vi "AlliGator 1-Exp + IRF Fit v2.vi"(0 "Decay":cluster{"t Array":dbl[], "Data Array":dbl[]}, 5 "IRF":cluster{"t Array":dbl[], "IRF Array":dbl[]}, 7 "Fit Options":T9={"Show Fit Residuals"=TRUE, "Fit Model"=enum."1-Exponential", "Residual Type"=enum."Standard", "Max Decay Percentile"=0.0, "Min Decay Percentile"=0.0, "Show Full Decay"=TRUE, "Weights"=enum."Unweighted", "Fitting Method"=enum."Least Square", "Compute Parameter Uncertainties"=TRUE, "Periodic Boundaries"=TRUE, "Model Calculation"=enum."Simulation", "Period"=1.2500000000000001e-08, "Termination Criteria"={"Max Iterations"=1000, "Max Function Calls"=0, "Max Time"=1000.0, "Function Tolerance"=1e-06, "Parameter Tolerance"=1e-06, "Gradient Tolerance"=0.0, "Min Lambda"=1e-06, "Max Lambda"=1e-06, "Initial Tick Count"=0}, "Offset Resolution"=1.2500000000000001e-08, "Use Local IRF"=TRUE, "Fitting Algorithm"=enum."Levenberg-Marquardt"} {"Offset Resolution" min=0.0; "Period" min=0.0; "Min Decay Percentile" min=0.0 max=1.0; "Max Decay Percentile" min=0.0 max=1.0}, 11 "error in (no error)":errorcluster, 12 "parameter bounds":T8) -> (4 "Fitted Decay":cluster{"t Array":dbl[], "Fitted Array":dbl[]}, 6 "Residuals":cluster{"t Array":dbl[], "Residual Array":dbl[]}, 8 "Fit Output":T2={"best nonlinear fit"=[], "best fit parameters"=[], "R^2"=0.0, "RMSE"=0.0, "error out"={"status"=FALSE, "code"=0, "source"=""}, "Fitting Method"=enum."Least Square", "number of function calls"=0, "number of iterations"=0, "covariance"=[], "Chi 2"=0.0, "DOF"=0, "Fit Convergence Criterion"=enum."Continue", "Fitting Algorithm"=enum."Levenberg-Marquardt", "Weighted Fit"=FALSE, "Gradient"=0.0, "|Delta Chi 2|"=0.0, "|Delta Chi 2|/Chi 2"=0.0, "Max |Delta a| /|a|"=0.0, "Lambda"=-1.0, "RSS"=0.0, "AIC"=0.0, "BIC"=0.0, "Max number of function calls"=0, "Max number of iterations"=0, "IRF"={"X Array"=[], "Y Array"=[]}, "IRF Normalization Factor"=0.0, "Decay Normalization Factor"=0.0}, 10 "Delta Best Fit Parameters":dbl[](array[numeric]), 13 "Guess Parameters Options":T1=enum."User-provided (normalized)", 14 "Guess Parameters":dbl[](array[numeric]), 15 "error out":errorcluster)   [LabVIEW 2021, in "AlliGator Decay Analysis.lvlib" / "AlliGator Decay Fit.lvlib"]
doc: "Legacy code for 1-Exp decay fit."
uses:
  AlliGator Decay Fit.lvlib
  Fits/IRF(X)PSED/Decay Fit Options v2.ctl
  Fits/Decay Convolution/Decay Model.ctl
  Fits/Residual Type.ctl
  Fits/IRF(X)PSED/Fit Weights Type.ctl
  Fits/Non-linear Fitting Method v2.ctl
  Fits/Fit Calculation Method.ctl
  Fits/Non-linear Fitting Algorithm.ctl
  Fits/Non-linear Fit Output v3.ctl
  Fits/Nonlinear Fit Method.ctl
  <vilib>/Analysis/Matrix/Datatypes/RealMatrix.ctl
  Fits/Convergence Criteria.ctl
  Graphs/XY Graph/XY Plot Data.ctl
  AlliGator Guess Parameters Options.ctl
  AlliGator Settings List.ctl
  Fits/Decay Convolution/Fit Control Data.ctl
  AlliGator Variables List.ctl
  Fits/Decay Convolution/LM model function and gradient (1-Exp, Convolved) v2.vi
  Phasor/Phasor Abort Parallel Computation.vi
  Fits/Decay Convolution/LM model function and gradient (1-Exp, Convolved, Periodic) v3.vi
  Fits/Decay Convolution/LM model function and gradient (1-Exp, Gated, Periodic).vi
  <vilib>/Utility/error.llb/Error Cluster From Error Code.vi
  Fits/Abort Fit Global.vi
  <vilib>/ErrorRing/Error Ring.xnode
  Time/Time.lvlib
  Fits/Fits.lvlib
  AlliGator Settings.lvlib
  Phasor/Phasor.lvlib
  AlliGator Globals, Variables & Constants.lvlib
  Error/Error.lvlib
  Graphs/XY Graph/XY Graph Add-Ons.lvlib
  <vilib>/Analysis/Matrix/NI_Matrix.lvlib
panel:
  out "CPU (s)":dbl
  out "XY Graph":T15(graph)
  # "Offset\nBaseline\nAmplitude\nLifetime"
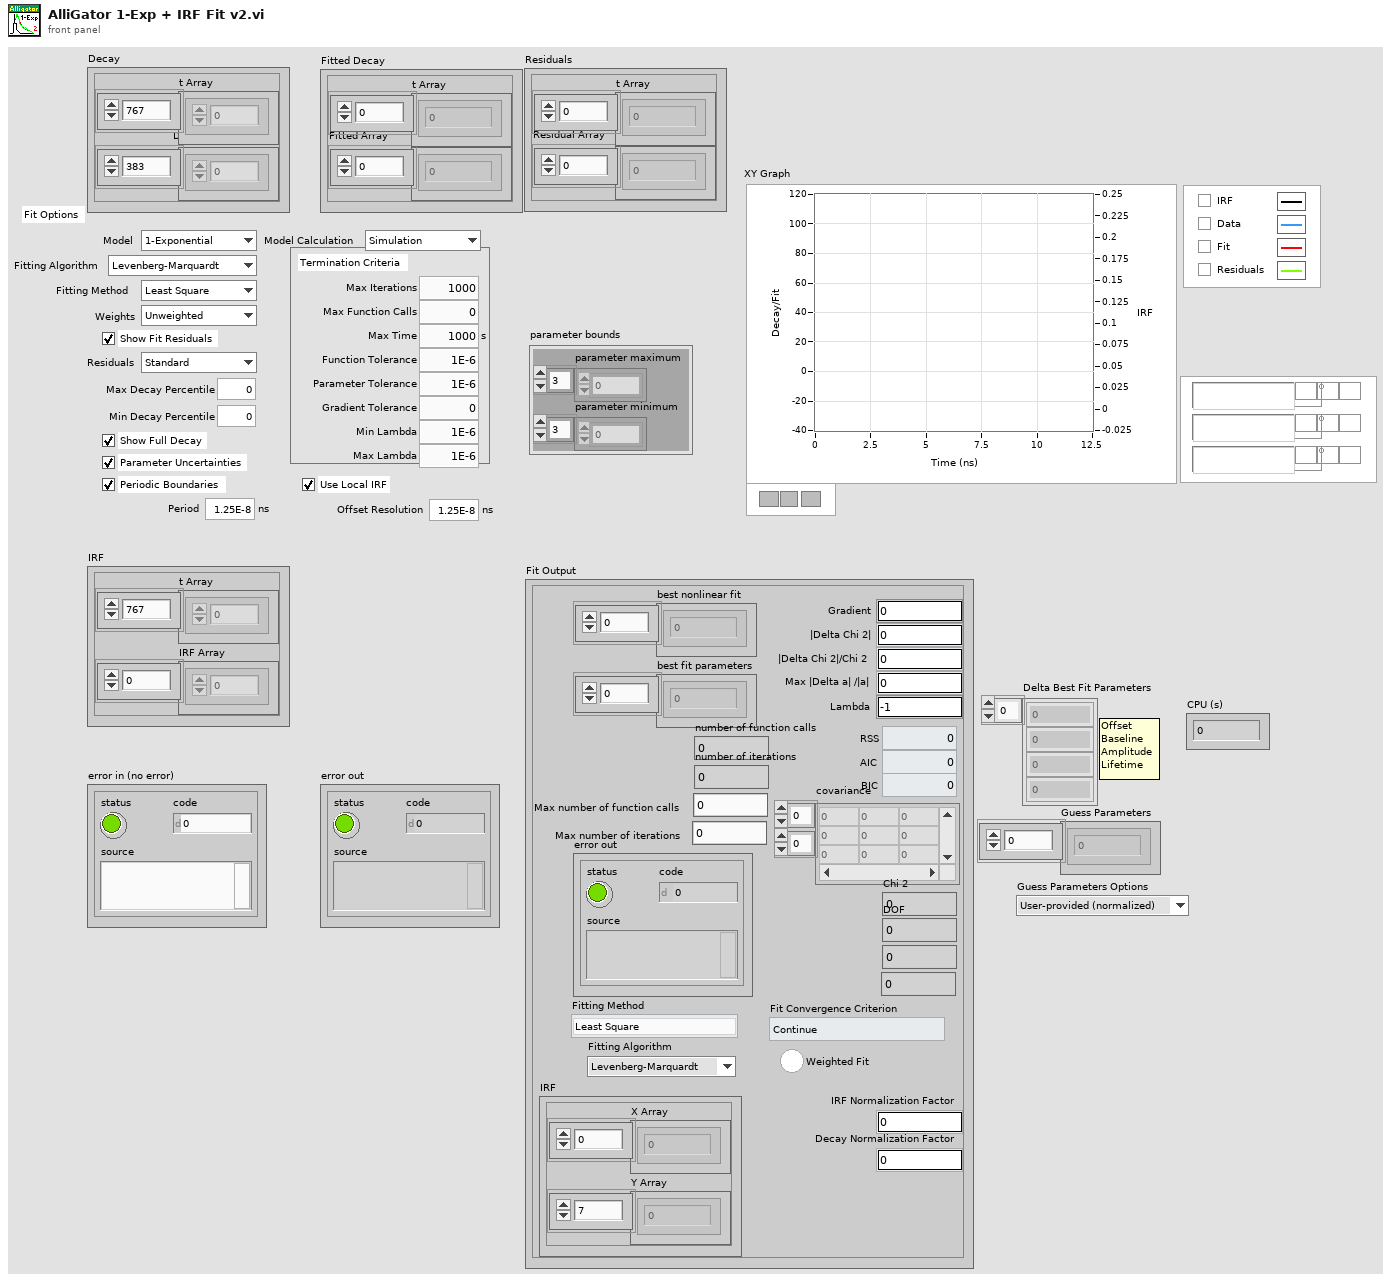
[diagram p1: front panel]
types:
  T1 = typedef "AlliGator Decay Analysis.lvlib/AlliGator Decay Fit.lvlib/AlliGator Guess Parameters Options.ctl" = enum16{"Numerically estimated", "User-provided", "User-provided (normalized)", "Last valid fitted parameters"}
  T2 = typedef "Fits.lvlib/Non-linear Fit Output v3.ctl" = cluster{"best nonlinear fit":dbl[], "best fit parameters":dbl[], "R^2":dbl, "RMSE":dbl, "error out":errorcluster, "Fitting Method":T3, "number of function calls":i32, "number of iterations":i32, "covariance":T4, "Chi 2":dbl, "DOF":i32, "Fit Convergence Criterion":T5, "Fitting Algorithm":T6, "Weighted Fit":bool, "Gradient":dbl, "|Delta Chi 2|":dbl, "|Delta Chi 2|/Chi 2":dbl, "Max |Delta a| /|a|":dbl, "Lambda":dbl, "RSS":dbl, "AIC":dbl, "BIC":dbl, "Max number of function calls":i32, "Max number of iterations":i32, "IRF":T7, "IRF Normalization Factor":dbl, "Decay Normalization Factor":dbl}
  T3 = typedef "Fits.lvlib/Nonlinear Fit Method.ctl" = enum16{"Least Square", "Least Absolute Residual", "Bisquare", "MLE"}
  T4 = typedef "NI_Matrix.lvlib/RealMatrix.ctl" = dbl[][]
  T5 = typedef "Fits.lvlib/Convergence Criteria.ctl" = enum16{"Continue", "Tolerances Exceeded", "Max Time Exceeded", "Max Iterations Exceeded", "Max Function Evaluations Exceeded", "Scale Range Exceeded"}
  T6 = typedef "Fits.lvlib/Non-linear Fitting Algorithm.ctl" = enum16{"Levenberg-Marquardt", "Trust-Region Dogleg"}
  T7 = typedef "XY Graph Add-Ons.lvlib/XY Plot Data.ctl" = cluster{"X Array":dbl[], "Y Array":dbl[]}
  T8 = cluster{"parameter minimum":dbl[], "parameter maximum":dbl[]}
  T9 = typedef "Fits.lvlib/Decay Fit Options v2.ctl" = cluster{"Show Fit Residuals":bool, "Fit Model":T10, "Residual Type":T11, "Max Decay Percentile":dbl, "Min Decay Percentile":dbl, "Show Full Decay":bool, "Weights":T12, "Fitting Method":T13, "Compute Parameter Uncertainties":bool, "Periodic Boundaries":bool, "Model Calculation":T14, "Period":dbl[unit], "Termination Criteria":cluster{"Max Iterations":i32, "Max Function Calls":i32, "Max Time":dbl[unit], "Function Tolerance":dbl, "Parameter Tolerance":dbl, "Gradient Tolerance":dbl, "Min Lambda":dbl, "Max Lambda":dbl, "Initial Tick Count":u32}, "Offset Resolution":dbl[unit], "Use Local IRF":bool, "Fitting Algorithm":T6}
  T10 = typedef "Fits.lvlib/Decay Model.ctl" = enum16{"1-Exponential", "2-Exponentials"}
  T11 = typedef "Fits.lvlib/Residual Type.ctl" = enum16{"Standard", "Normalized", "Reduced"}
  T12 = typedef "Fits.lvlib/Fit Weights Type.ctl" = enum16{"Unweighted", "1/Variance", "Best of All"}
  T13 = typedef "Fits.lvlib/Non-linear Fitting Method v2.ctl" = enum16{"Least Square", "Least Absolute Residual", "Bisquare", "MLE", "-", "Best of All"}
  T14 = typedef "Fits.lvlib/Fit Calculation Method.ctl" = enum16{"Simulation", "Convolution", "Integration"}
  T15 = cluster{"t Array":dbl[], "best nonlinear fit":dbl[]}[]
  T16 = typedef "AlliGator Settings.lvlib/AlliGator Settings List.ctl" = enum16{"GUI:Visible Settings Tab", "GUI:Last Run Version", "Source Image:Use Image Histogram for Contrast", "Source Image:Low Count Pixels Rejection Options", "Source Image:High Count Pixels Rejection Options", "Source Image:Use Image Brightness", "Source Image:Blend Overlay with Image Background", "Source Image:Use Fixed ROI Diameter", "Source Image:ROI Diameter", "Source Image:ROI Center Color", "Source Image:Peak Threshold", "Source Image:Intensity Threshold", "Source Image:Image Binning Options", "Source Image:Image Smoothing Options", "Source Image:Image Histogram Active", "Source Image:Invert Binary Mask", "Source Image:Hot Pixel Removal", "Source Image:Overlay Analyzed ROI Center", "Source Image:Auto-Adjust Contrast", "Source Image:Histogram Lower Percentile", "Source Image:Histogram Upper Percentile", "Source Image:Save Source Image", "Source Image:Scale Bar Options", "Source Image:Image Resolution (Pixel Size)", "Source Image:Flatfield Correction", "Source Image:Show Dead Left Columns Correction", "Source Image:Dead Left Columns Correction", "Source Image:Image Pre-Processing Operations Order", "Source Image:Overlay ROI Median", "Source Image:Median Overlay Color", "Data Information:Gate Width", "Data Information:Nanotime Gate Separation", "Data Information:Macrotime Gate Separation", "Data Information:Gate Step", "Data Information:# Gates", "Data Information:Gate Image Exposure", "Data Information:Gate Image Integration", "Data Information:Gates to Skip", "Data Information:Gates to Keep", "Data Information:Define Gates to", "Data Information:Channel Name", "Data Information:Available Channel Names", "Data Information:Channel Arithmetic", "Data Information:Background File Subtraction", "Data Information:Background File", "Data Information:Background Scaling Factor", "Data Information:Background Pile-up Correction", "Data Information:Background Pixel Well Capacity", "Data Information:Laser Period", "Data Information:SYNC Period", "Data Information:Pile-up Correction", "Data Information:Pixel Well Capacity", "Data Information:Dataset Scaling Factor", "Fluorescence Decay_Decay Pre-Processing:Reverse Gates", "Fluorescence Decay_Decay Pre-Processing:Verbose Decay Pre-Processing", "Fluorescence Decay_Decay Pre-Processing:Use Decay Pre-Processing", "Fluorescence Decay_Decay Pre-Processing:Background Subtraction", "Fluorescence Decay_Decay Pre-Processing:Background Definition Range", "Fluorescence Decay_Decay Pre-Processing:Baseline Subtraction Method", "Fluorescence Decay_Decay Pre-Processing:Decay Pre-Processing Operations Order", "Fluorescence Decay_Decay Pre-Processing:Smoothing Parameter", "Fluorescence Decay_Decay Pre-Processing:Shift Decay", "Fluorescence Decay_Decay Pre-Processing:Decay Shift Parameters", "Fluorescence Decay_Decay Pre-Processing:Fold Decay", "Fluorescence Decay_Decay Pre-Processing:# Folds", "Fluorescence Decay_Decay Pre-Processing:1-Normalize Decay", "Fluorescence Decay_Decay Pre-Processing:[0-1]-Normalize Decay", "Fluorescence Decay_Decay Pre-Processing:Smoothen Decay", "Fluorescence Decay_Decay Pre-Processing:Extrapolate Decay", "Fluorescence Decay_Decay Pre-Processing:Use Periodicity", "Fluorescence Decay_Decay Pre-Processing:Use Cursors", "Fluorescence Decay_Decay Pre-Processing:Tail Fraction", "Fluorescence Decay_Decay Pre-Processing:Head Fraction", "Fluorescence Decay_Decay Pre-Processing:Additional Points", "Fluorescence Decay_Decay Pre-Processing:Straighten Decay", "Fluorescence Decay_Decay Pre-Processing:Constant Background", "Fluorescence Decay_Decay Pre-Processing:Pixel-Normalize Decay", "Fluorescence Decay_Advanced Analysis:Extract IRF instead of Decay", "Fluorescence Decay_Advanced Analysis:IRF Extraction Options", "Fluorescence Decay_Advanced Analysis:IRF Optimization Options", "Fluorescence Decay_Advanced Analysis:Square Pulse Options", "Fluorescence Decay_Advanced Analysis:IRF Order", "Fluorescence Decay_Advanced Analysis:IRF Time Constants", "Fluorescence Decay_Advanced Analysis:Wavelet Analysis Options", "Fluorescence Decay_Advanced Analysis:Average Lifetime Options", "Fluorescence Decay_Fit Options:Fit Options", "Fluorescence Decay_Fit Options:Use Legacy Fitting Approach", "Fluorescence Decay_Fit Options:Use Data Information Laser Period", "Fluorescence Decay_Fit Parameters:Displayed Fit Parameters", "Fluorescence Decay_Fit Parameters:Fit Parameter Constraints", "Fluorescence Decay_Fit Parameters:Export Tabulated Results", "Fluorescence Decay_Fit Parameters:MLE Baseline Offset Type", "Fluorescence Decay_Fit Parameters:MLE Baseline Offset", "Fluorescence Decay_Fit Parameters:Guess Parameter Names", "Fluorescence Decay_Fit Parameters:Guess Parameter Values", "Fluorescence Decay_Fit Parameters:Guess Parameters Options", "Fluorescence Decay_Styles:Show Last Decay Only", "Fluorescence Decay_Styles:Decay Graph Color Array", "Fluorescence Decay:Decay Graph Active", "Fluorescence Decay Statistics:Min Peak Value", "Fluorescence Decay Statistics:Reject Low Decay Peak Pixels", "Fluorescence Decay Statistics:Reject High Decay Peak Pixels", "Fluorescence Decay Statistics:Max Peak Value", "Time Traces:Use File Timestamp", "Time Traces:Time Step", "Time Traces:Use Intensity Correction File", "Time Traces:Intensity Correction File", "Phasor Plot:Phasor Plot Smoothing Options", "Phasor Plot:Phasor Plot Size", "Phasor Plot:Phasor Plot Graphics Options", "Phasor Plot:Cumulative Phasor Plot", "Phasor Plot:Use Phasor Brightness", "Phasor Plot:Blend Overlay with Phasor Background", "Phasor Plot:Save Phasor Plot", "Phasor Plot:Show References", "Phasor Plot:Phasor Ratio Decay Range", "Phasor Plot:Exponential Fading", "Phasor Plot:Phasor Ratio Reference Colors", "Phasor Plot:Reference Radius", "Phasor Plot:Show Color Map Vertices", "Phasor Plot:Phasor Plot Active", "Phasor Plot:Phasor Ratio Color Map Type", "Phasor Plot:Phasor Ratio Color Map", "Phasor Plot:Phasor Ratio Display Range", "Phasor Plot:Selected Image ROI(s)", "Phasor Plot:All Image ROIs", "Phasor Plot:Selected Phasor Plot ROI(s)", "Phasor Plot:All Phasor Plot ROIs", "Phasor Plot:Phasor Ratio Color-Coded Quantity", "Phasor Plot:Store Phasor Harmonics", "Phasor Plot:Draw Reference Segment", "Phasor Plot:User-Defined Quantity", "Phasor Graph:Phasor Frequency", "Phasor Graph:Phasor Ratio Type", "Phasor Graph:Pixel-level Phasor Computation", "Phasor Graph:Save Phasor Graph", "Phasor Graph:Phasor Graph Active", "Phasor Graph:Phasor SDV Options", "Phasor Calibration:Use Backup Calibration if needed", "Phasor Graph:Define Shortest Lifetime as", "Phasor Calibration:Backup Calibration Type", "Phasor Calibration:Calibration Type", "Phasor Calibration:Calibration Lifetime", "Phasor Calibration:Calibration Map Algorithm", "Single-Exponential Phasor Locus (SEPL):Gate Parameters", "Single-Exponential Phasor Locus (SEPL):User-defined Gate", "Single-Exponential Phasor Locus (SEPL):User-defined IRF", "Single-Exponential Phasor Locus (SEPL):Phasor Parameters", "Single-Exponential Phasor Locus (SEPL):Decay & IRF Parameters", "Single-Exponential Phasor Locus (SEPL):Display Parameters", "Lifetime Analysis:Decay Analysis Parameters", "Lifetime Analysis:Lifetime Map Active", "Plugins:Python Settings", "Miscellaneous:Verbose Mode", "Miscellaneous:Beep after Script", "Miscellaneous:Saved Image File Format", "Miscellaneous:Exported Gate Image Settings", "Miscellaneous:Include Loading in Timing", "Miscellaneous:Verbose Settings Mode", "Miscellaneous:Histogram Options", "Miscellaneous:Beep on Error", "Miscellaneous:# Logical Processors Used", "Miscellaneous:ROI Description Max Characters", "Miscellaneous:Verbose Error Mode", "Miscellaneous:Transparent Mask Color"}
  T17 = typedef "Fits.lvlib/Fit Control Data.ctl" = cluster{"IRF":T7, "Laser Period":dbl, "SYNC Period":dbl}
  T18 = typedef "Fits.lvlib/Decay Fit Parameters In List.ctl" = enum16{"Offset", "Baseline", "A_1", "tau_1", "A_2", "tau_2"}
  T19 = typedef "Fits.lvlib/Fit Results (statistics).ctl" = cluster{"Chi2/DOF":dbl, "R2":dbl, "RMSE":dbl, "Fitting Method":T13, "Fitting Algorithm":T6}
  T20 = typedef "AlliGator Globals, Variables & Constants.lvlib/AlliGator Variables List.ctl" = enum16{"---- GUI ----", "GUI:Initialization Status", "GUI:State Indicators Refnum", "GUI:Original AlliGator Menu Items", "GUI:Current Action Loop State", "GUI:Script in progress", "GUI:Playback", "GUI:Loop Playback", "GUI:Search ROI Used", "GUI:Search ROI", "Decay Graph Max Legend Size", "Intensity Graph Max Legend Size", "Decay Statistics Graph Max Legend Size", "Phasor Graph Max Legend Size", "Phasor Ratio Graph Max Legend Size", "Lifetime Graph Max Legend Size", "---- Files ----", "Files:Export Dataset Frames as Individual Files", "Files:Show Batch Export Help Balloons", "Files:Frames in Dataset", "Files:ptu File Frame Start Indices", "Files:Current Frame in Dataset", "Files:Current Frame Timestamp", "Files:Dataset Loaded", "Files:Dataset Metadata", "Files:Dataset Channel", "Files:Dataset Data Description", "Files:Background Dataset Metadata", "Files:Background Dataset Channel", "Files:Background Dataset Data Description", "Files:Background File Subtraction", "Files:Background File Path", "Files:Background File Pile-up Correction", "Files:Background File Pixel Well Capacity", "Files:Background File Scaling Factor", "Files:Current Dataset Load Settings", "Files:Dataset Path", "Files:ICCD-specific Information", "Files:Macrotime Gate Separation", "------ Python Plugins ------", "Python Plugins:Information", "Python Plugins:Python Session", "Python Plugins:Valid Python Session?", "---- Source Image ----", "Source Image:ROIs", "Source Image:Current ROI", "Source Image:ROI Event Refnum", "X_Source Image Display Range", "X_Source Image Palette Information", "X_Type of Displayed Image", "X_Time Gate Slider", "Source Image:Palette List", "Source Image:Scale", "Source Image:ROI Overlay Color", "Source Image:Overlay to Erase", "Source Image:Is Displayed Image Accumulated", "Source Image:White Light Image Modified", "Source Image:Mask Image Modified", "---- Image Profile Window ----", "Image Profile:Window Event Refnum", "Image Profile:IntensityType", "Image Profile:Intensity Average Type", "Image Profile:Intensity-weighted SDV", "Image Profile:Box Profile Type", "Image Profile:Window Open", "Image Profile:Plotted Fit Parameter", "------ Phasor Graph -------", "Phasor Graph:Show Line", "---- Phasor Plot ---", "Phasor Plot:Parameters Changed", "Phasor Plot:FLI Dataset Modified since last Calculation", "Phasor Harmonics Data", "Selected Phasor Harmonics", "Phasor Harmonic Manager Event Refnum", "Phasor Plot:ROIs", "Phasor Plot:Current ROI", "Phasor Plot:ROI Event Refnum", "Phasor Plot:Image Reference Points", "Phasor Plot:Computed", "Phasor Plot:Palette Information", "Phasor Plot:Palette List", "Phasor Plot:Phasor Ratio Palette Information", "Phasor Plot:Phasor Ratio Palette List", "Phasor Plot:Image Scale", "Phasor Plot:Image Overlay to Erase", "Phasor Plot:Image Elements to Update", "Phasor Plot:Current Calculation Parameters", "Phasor Plot:Current Calibration Options", "Phasor Plot:Reset Cumulated Phasor Plot", "Phasor Plot:Reference 1", "Phasor Plot:Lifetime Reference 1", "Phasor Plot:Reference 1 Frequency", "Phasor Plot:Reference 2", "Phasor Plot:Lifetime Reference 2", "Phasor Plot:Reference 2 Frequency", "---- Decay Analysis ----", "Number of Selected Decays to Fit", "LS Fit Results", "LAR Fit Results", "BS Fit Results", "Last Decay Max - Min", "Best Fit Parameters", "Best Fit Parameter Names", "Actual Size X", "Actual Size Y", "Binning X", "Binning Y", "Actual # Gates", "Dataset Number", "Gates to...", "Gates Skipped", "Gates to keep", "Gate Step", "Gate Separation", "Reversed Gates", "Pile-up Correction", "Pixel Well Capacity", "Background Subtracted", "Background Subtraction Method", "Background Definition Range", "Background File (deprecated)", "Number of Dataset Accumulated", "Array of Accumulated Dataset Paths", "Do Averaged Datasets", "Destination File Path", "Process Plot Target", "Use 1/D as Phasor Frequency", "---- Decay Fit Parameter Map -----", "Decay Fit Parameter Map:Palette Information", "Decay Fit Parameter Map:Palette List", "------- Local Decay Window ---------", "Local Decay Graph Window:Event Refnum", "Local Decay Graph Window:Use normalized IRF for convolution", "----- Miscellaneous ----", "Misc:Skippable Dialog Windows Status"}
  T21 = cluster{"t Array":dbl[], "best nonlinear fit":dbl[]}
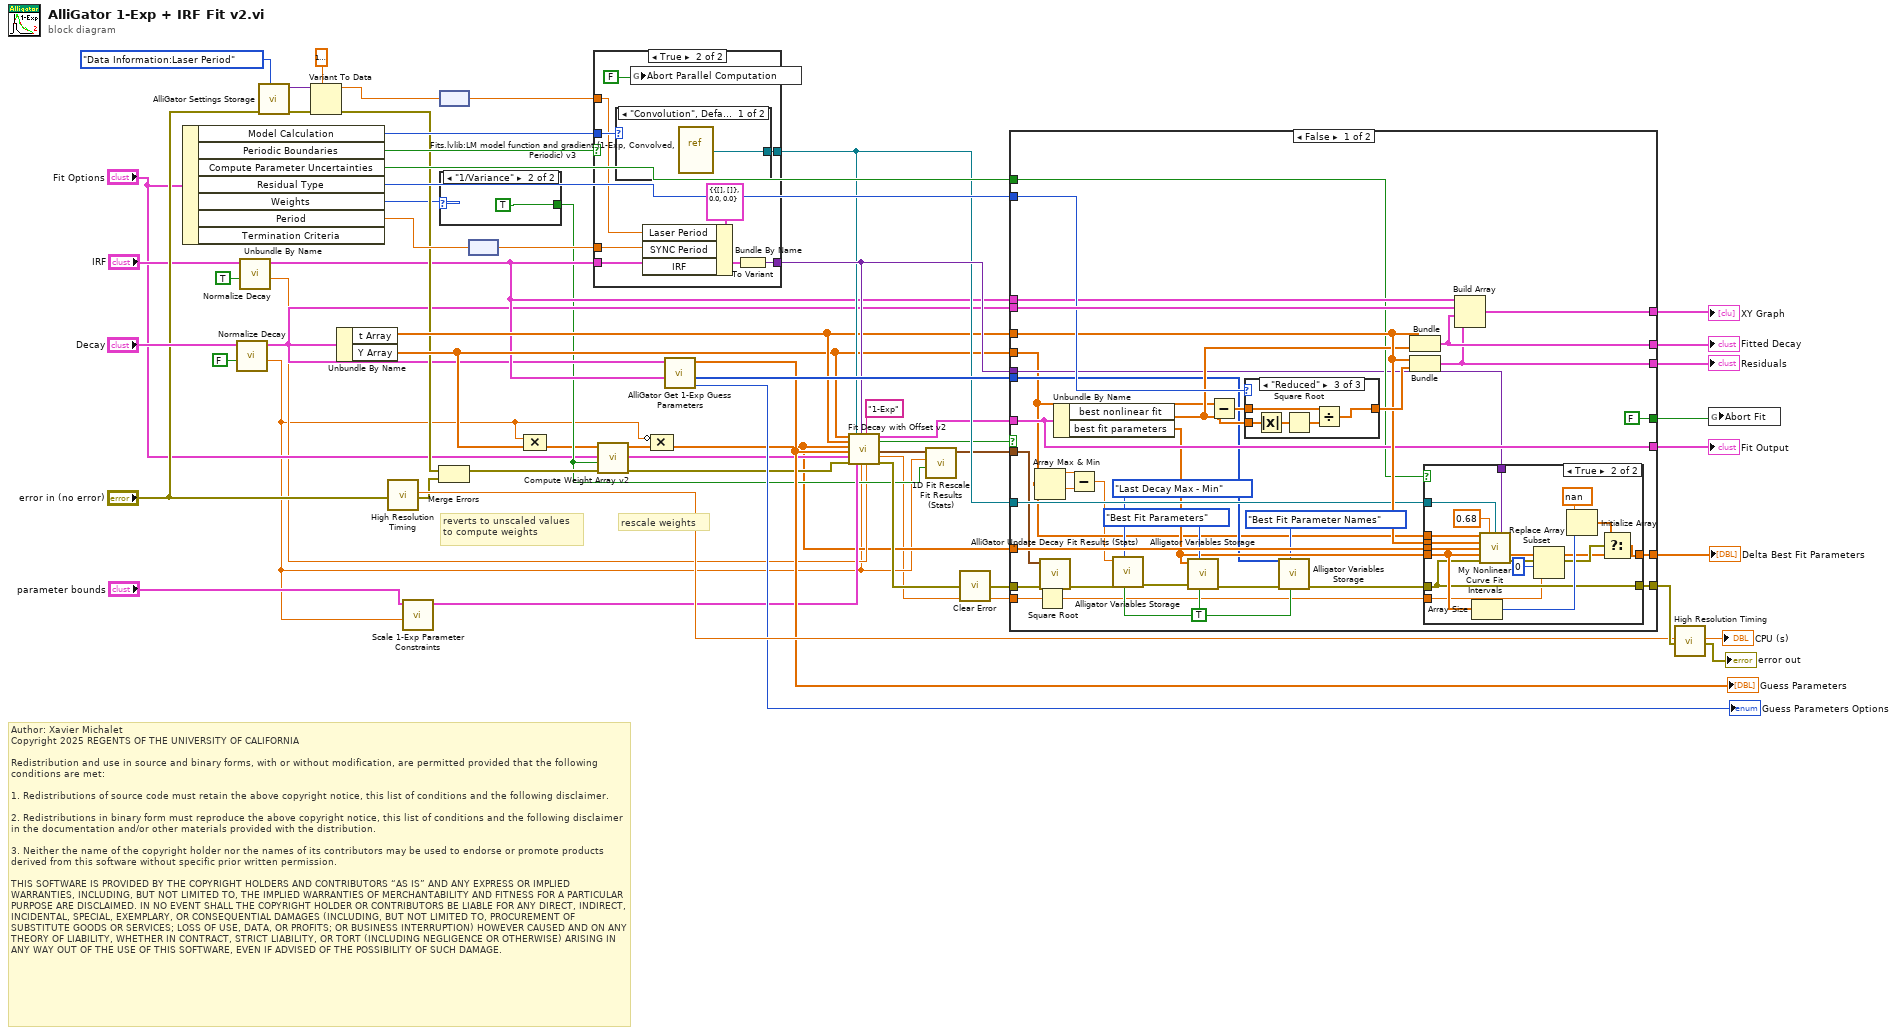
[diagram p0: block diagram]
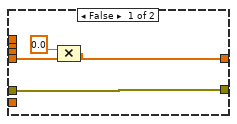
[diagram p3: hidden frame]
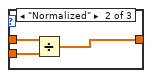
[diagram p5: hidden frame]
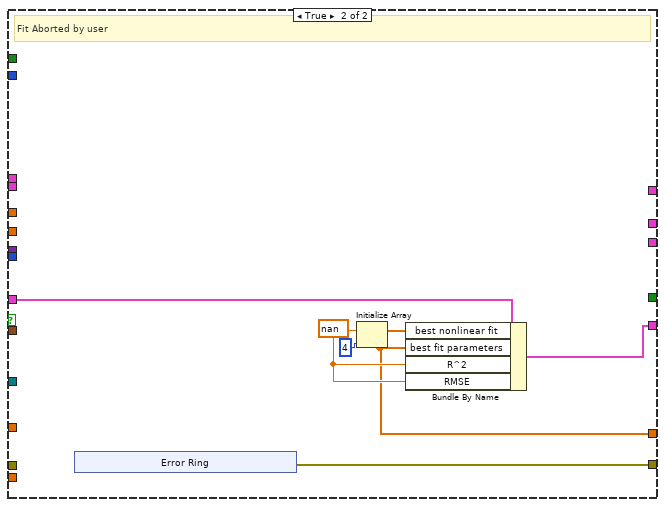
[diagram p6: hidden frame]
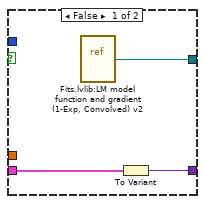
[diagram p7: hidden frame]
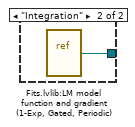
[diagram p8: hidden frame]
diagram:
  # "Author: Xavier Michalet\nCopyright 2025 REGENTS OF THE UNIVERSITY OF CALIFORNIA\n\nRedistribution and use in source and binary forms, with or without modification, are permitted provided that the following conditions are met:\n\n1. Redistributions of source code must retain the above copyright notice, this list of conditions and the following disclaimer.\n\n2. Redistributions in binary form must reproduce the above copyright notice, this list of conditions and the following disclaimer in the documentation and/or other materials provided with the distribution.\n\n3. Neither the name of the copyright holder nor the names of its contributors may be used to endorse or promote products derived from this software without specific prior written permission.\n\nTHIS SOFTWARE IS PROVIDED BY THE COPYRIGHT HOLDERS AND CONTRIBUTORS “AS IS” AND ANY EXPRESS OR IMPLIED WARRANTIES, INCLUDING, BUT NOT LIMITED TO, THE IMPLIED WARRANTIES OF MERCHANTABILITY AND FITNESS FOR A PARTICULAR PURPOSE ARE DISCLAIMED. IN NO EVENT SHALL THE COPYRIGHT HOLDER OR CONTRIBUTORS BE LIABLE FOR ANY DIRECT, INDIRECT, INCIDENTAL, SPECIAL, EXEMPLARY, OR CONSEQUENTIAL DAMAGES (INCLUDING, BUT NOT LIMITED TO, PROCUREMENT OF SUBSTITUTE GOODS OR SERVICES; LOSS OF USE, DATA, OR PROFITS; OR BUSINESS INTERRUPTION) HOWEVER CAUSED AND ON ANY THEORY OF LIABILITY, WHETHER IN CONTRACT, STRICT LIABILITY, OR TORT (INCLUDING NEGLIGENCE OR OTHERWISE) ARISING IN ANY WAY OUT OF THE USE OF THIS SOFTWARE, EVEN IF ADVISED OF THE POSSIBILITY OF SUCH DAMAGE."
  # "rescale weights"
  # "reverts to unscaled values to compute weights"
  n1 = Unbundle By Name("Fit Options") -> ("Model Calculation"=w40:T14, "Periodic Boundaries"=w47:bool, "Compute Parameter Uncertainties"=w48:bool, "Residual Type"=w51:T11, "Weights"=w18:T12, "Period"=w37:dbl[unit])  [unwired: 1 out]
  n2 = call "Normalize Decay.vi"("IRF (F)"=FALSE, "Decay"="Decay") -> ("Normalization Factor"=w2:dbl, "Normalized Decay"=w17:cluster{"t Array":dbl[], "Y Array":dbl[]})  [unwired: 7 in, 1 out]
  n3 = call "Normalize Decay.vi"("IRF (F)"=TRUE, "Decay"="IRF") -> ("Normalization Factor"=w5:dbl, "Normalized Decay"=w19:cluster{"t Array":dbl[], "Y Array":dbl[]})  [unwired: 7 in, 1 out]
  n4 = call "AlliGator Settings Storage.vi"("AlliGator Settings List"=AlliGator_Settings_List."Data Information:Laser Period", "Error In"="error in (no error)") -> ("Error Out"=w44:errorcluster, "Variant Data out"=w45:variant)  [unwired: 8 in]
  n5 = Variant To Data(error in=w44, type=dbl[unit] 1e-09 ("New"), Variant=w45) -> (data=w42:dbl[unit], error out=w25:errorcluster)
  n6 = Unbundle By Name(w17) -> ("t Array"=w33:dbl[], "Y Array"=w30:dbl[])
  n7 = call "High Resolution Timing.vi"("Error In"="error in (no error)") -> ("elapsed (relative) seconds"=w53:dbl, "Error Out"=w27:errorcluster)  [unwired: 16 in, 1 out]
  n8 = call "Scale 1-Exp Parameter Constraints.vi"("Normalization Factor"=w2, "parameter bounds in"="parameter bounds") -> ("parameter bounds out"=w10:T8)  [unwired: 9 in]
  n9 = Merge Errors(w25, w27) -> (w24:errorcluster)
  n10 = node(w42) -> (w41:dbl)
  n11 = case shown="\"1/Variance\"" w18 {
    tunnel: [_ TRUE ("Weighted Fit")] -> w8
    frame "Unweighted", Default {
    }
    frame "1/Variance" {
    }
  }
  n12 = node(w37) -> (w36:dbl)
  n13 = Compound Arithmetic op=MULTIPLY(w2, w30) -> (w4:dbl[])
  n14 = case shown="True" w47 {
    tunnel: [w62 w71] -> w34
    tunnel: w19 -> [w61 w70]
    tunnel: [w60 w68] -> w35
    tunnel: w41 -> [_ w64]
    tunnel: w40 -> [_ w66]
    tunnel: w36 -> [_ w63]
    frame False {
      n15 = vi-ref "Fits.lvlib:LM model function and gradient (1-Exp, Convolved) v2.vi"() -> (w62:refnum<vi>)
      n16 = To Variant(anything=w61) -> (Variant=w60:variant)
    }
    frame True {
      n17 = case shown="\"Convolution\", Default" w66 {
        tunnel: [w72 w73] -> w71
        frame "Convolution", Default {
          n18 = vi-ref "Fits.lvlib:LM model function and gradient (1-Exp, Convolved, Periodic) v3.vi"() -> (w72:refnum<vi>)
        }
        frame "Integration" {
          n19 = vi-ref "Fits.lvlib:LM model function and gradient (1-Exp, Gated, Periodic).vi"() -> (w73:refnum<vi>)
        }
      }
      n20 = global write "Phasor Abort Parallel Computation.vi" "Abort Parallel Computation"(FALSE ("Abort Parallel Computation")) -> ()
      n21 = Bundle By Name(cluster=T17 {"IRF"={"X Array"=[], "Y Array"=[]}, "Laser Period"=0.0, "SYNC Period"=0.0}, "Laser Period"=w64, "SYNC Period"=w63, "IRF"=w70) -> (w69:T17)
      n22 = To Variant(anything=w69) -> (Variant=w68:variant)
    }
  }
  n23 = call "Compute Weight Array v2.vi"("Error In"=w24, "Weighted Fit"=w8, "Data Array"=w4) -> ("Error Out"=w26:errorcluster, "Weight Array"=w31:dbl[])  [unwired: 7 in]
  n24 = Compound Arithmetic op=MULTIPLY(invert w2, w31) -> (w3:dbl[])
  n25 = call "AlliGator Get 1-Exp Guess Parameters.vi"("IRF"=w19, "Decay"=w17) -> ("Guess Parameters Type"=→"Guess Parameters Options":T1, "Guess Parameters Names"=w39:T18[], "Guess Parameters"=w32:dbl[])  [unwired: 7 in]
  "Guess Parameters" <- w32
  n26 = call "Fit Decay with Offset v2.vi"("Y Array"=w30, "X Array"=w33, "Weights"=w3, "Initial Parameters"=w32, "Decay Fit Options"="Fit Options", "error in (no error)"=w26, "f(x,a)"=w34, "parameter bounds"=w10, "Data"=w35, "Decay Normalization Factor"=w2, "Model Name"="1-Exp", "IRF Normalization Factor"=w5) -> ("Fit Output"=w11:T2, "Fit Aborted?"=w23:bool, "Fit Results (Stats)"=w13:T19[], "C_00"=w1:dbl, "error out"=w21:errorcluster)  [unwired: 3 in]
  n27 = call "1D Fit Rescale Fit Results (Stats).vi"("Weighted"=w8, "Normalization Factor"=w2, "Fit Results (Stats) in"=w13) -> ("Fit Results (Stats) out"=w12:T19[])  [unwired: 8 in]
  n28 = call "Clear Error.vi"("Error In"=w21) -> ("no Error Out"=w20:errorcluster)  [unwired: 8 in]
  n29 = case shown="False" w23 {
    tunnel: w17 -> [w109 _]
    tunnel: [w108 _] -> w58
    tunnel: [w107 _] -> w57
    tunnel: [w106 w144] -> w56
    tunnel: [w105 w140] -> w55
    tunnel: [w104 _] -> w54
    tunnel: w51 -> [w103 _]
    tunnel: w33 -> [w100 _]
    tunnel: w34 -> [w99 _]
    tunnel: w30 -> [w81 _]
    tunnel: w3 -> [w98 _]
    tunnel: w19 -> [w97 _]
    tunnel: w11 -> [w95 w143]
    tunnel: [w95 w142] -> w49
    tunnel: w48 -> [w94 _]
    tunnel: w35 -> [w93 _]
    tunnel: w39 -> [w87 _]
    tunnel: w20 -> [w86 _]
    tunnel: w12 -> [w77 _]
    tunnel: [FALSE ("Abort Fit") _] -> w7
    tunnel: w1 -> [w75 _]
    frame False {
      w83 = TRUE ("Get(F)/Set")
      n30 = Array Max & Min(array=w81) -> (max value=w80:dbl, min value=w79:dbl)  [unwired: 2 out]
      n31 = Square Root(x=w75) -> (sqrt(x)=w74:dbl)
      n32 = call "AlliGator Update Decay Fit Results (Stats).vi"("error in (no error)"=w86, "Fit Results"=w77) -> ("error out"=w85:errorcluster)  [unwired: 9 in]
      n33 = Unbundle By Name(w95) -> ("best nonlinear fit"=w96:dbl[], "best fit parameters"=w91:dbl[])
      n34 = Subtract(x=w80, y=w79) -> (x-y=w78:dbl)
      n35 = call "Alligator Variables Storage.vi"("Get(F)/Set"=w83, "AlliGator Variable"=AlliGator_Variables_List."Last Decay Max - Min" ("Alligator Variable"), "Error In"=w85, "Data in"=w78) -> ("Error Out"=w84:errorcluster)  [unwired: 5 in, 2 out]
      n36 = call "Alligator Variables Storage.vi"("Get(F)/Set"=w83, "AlliGator Variable"=AlliGator_Variables_List."Best Fit Parameters" ("Alligator Variable"), "Error In"=w84, "Data in"=w91) -> ("Error Out"=w90:errorcluster)  [unwired: 5 in, 2 out]
      n37 = Subtract(x=w81, y=w96) -> (x-y=w102:dbl[])
      n38 = case shown="\"Reduced\"" w103 {
        tunnel: w102 -> [w131 w134 w139]
        tunnel: [w131 w132 w137] -> w101
        tunnel: w96 -> [_ w133 w138]
        frame "Standard", Default {
        }
        frame "Normalized" {
          n39 = Divide(x=w134, y=w133) -> (x/y=w132:dbl[])
        }
        frame "Reduced" {
          n40 = Absolute Value(x=w138) -> (abs(x)=w136:dbl[])
          n41 = Square Root(x=w136) -> (sqrt(x)=w135:dbl[])
          n42 = Divide(x=w139, y=w135) -> (x/y=w137:dbl[])
        }
      }
      n43 = call "Alligator Variables Storage.vi"("Get(F)/Set"=w83, "AlliGator Variable"=AlliGator_Variables_List."Best Fit Parameter Names" ("Alligator Variable"), "Error In"=w90, "Data in"=w87) -> ("Error Out"=w89:errorcluster)  [unwired: 5 in, 2 out]
      n44 = Bundle("t Array"=w100, "best nonlinear fit"=w96) -> (w107:T21)  [unwired: 1 in]
      n45 = Bundle("t Array"=w100, w101) -> (w104:cluster{"t Array":dbl[], dbl[]})  [unwired: 1 in]
      n46 = case shown="True" w94 {
        tunnel: [w113 w117] -> w106
        tunnel: [w111 w118] -> w105
        tunnel: w100 -> [_ w129]
        tunnel: w99 -> [_ w128]
        tunnel: w98 -> [_ w127]
        tunnel: w93 -> [_ w126]
        tunnel: w91 -> [w112 w124]
        tunnel: w81 -> [_ w125]
        tunnel: w89 -> [w113 w117]
        tunnel: w74 -> [_ w114]
        frame False {
          n47 = Compound Arithmetic op=MULTIPLY(0.0, w112) -> (w111:dbl[])
        }
        frame True {
          n48 = Array Size(array=w124) -> (size(s)=w123:i32)
          n49 = call "My Nonlinear Curve Fit Intervals.vi"("Y"=w125, "confidence level"=0.68, "f(x,a)"=w128, "data"=w126, "X"=w129, "Weight"=w127, "best fit parameters"=w124, "error in (no error)"=w117) -> ("delta best fit parameters"=w119:dbl[], "error out"=w120:errorcluster)  [unwired: 6 in]
          n50 = Replace Array Subset(array=w119, new element=w114, index=0) -> (w116:dbl[])
          n51 = Initialize Array(nan ("element"), w123) -> (w121:dbl[])
          n52 = Select(t=w121, s=w120, f=w116) -> (s? t:f=w118:dbl[])
        }
      }
      n53 = Build Array(w97, w109, w107, w104) -> (w108:T15)
    }
    frame True {
      w141 = nan ("element")
      # "Fit Aborted by user"
      n54 = xnode "Error Ring"() -> ("error out"=w144:errorcluster)
      n55 = Initialize Array(w141, 4 ("dimension size")) -> (w140:dbl[])
      n56 = Bundle By Name(cluster=w143, "best nonlinear fit"=w140, "best fit parameters"=w140, "R^2"=w141, "RMSE"=w141) -> (w142:T2)
    }
  }
  "Fitted Decay" <- w57
  "XY Graph" <- w58
  "Delta Best Fit Parameters" <- w55
  "Residuals" <- w54
  "Fit Output" <- w49
  n57 = call "High Resolution Timing.vi"("relative seconds (NaN)"=w53, "Error In"=w56) -> ("elapsed (relative) seconds"=→"CPU (s)":dbl, "Error Out"=→"error out":errorcluster)  [unwired: 15 in, 1 out]
  n58 = global write "Abort Fit Global.vi" "Abort Fit"(w7) -> ()
